vi "DisconnectCameraRslt.vi"(8 "error in (no error)":errorcluster, 11 "CameraTestingUI in":refnum<class "CameraTestingUI.lvclass">) -> (0 "error out":errorcluster, 3 "CameraTestingUI out":refnum<class "CameraTestingUI.lvclass">)   [LabVIEW 2020, in "CameraTestingUI.lvlib" / "CameraTestingUI.lvclass"]
uses:
  CameraTestingUI.lvclass
  CameraTestingUI.lvclass/CameraTestingUI.ctl
  Private/TypeDef/ConnectionStatus.ctl
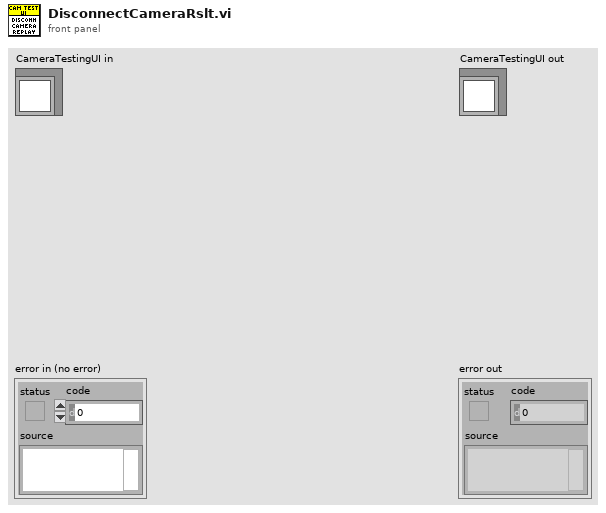
[diagram p1: front panel]
types:
  T1 = enum8{"Enabled", "Disabled", "Disabled and Grayed Out"}
  T2 = typedef "CameraTestingUI.lvlib/CameraTestingUI.lvclass/ConnectionStatus.ctl" = u16
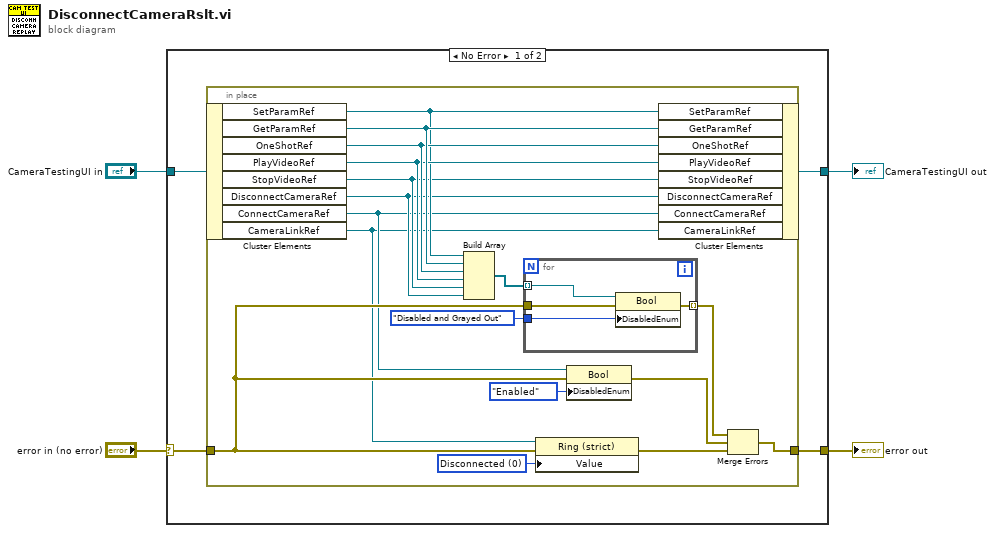
[diagram p0: block diagram]
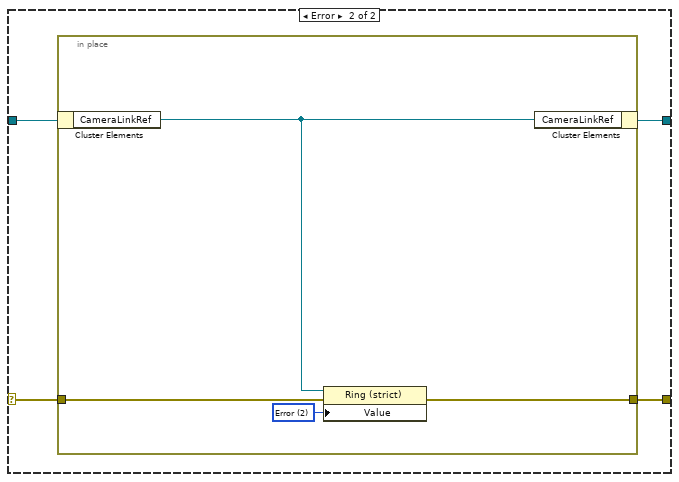
[diagram p2: hidden frame]
diagram:
  n1 = case shown="No Error" "error in (no error)" {
    selector: "error in (no error)" -> [w6 w32]
    tunnel: "CameraTestingUI in" -> [w8 w33]
    tunnel: [w7 w30] -> w3
    tunnel: [w5 w31] -> w1
    frame No Error {
      n2 = in-place {
        in-place-border: w6 -> [w17]
        in-place-border: [w13] -> w5
        w9 = T2 0 items=["Disconnected", "Connected", "Error"] ("Value")
        n3 = in-place-cluster #1(w8) -> ("SetParamRef"=w22:refnum<vi>, "GetParamRef"=w25:refnum<vi>, "OneShotRef"=w24:refnum<vi>, "PlayVideoRef"=w23:refnum<vi>, "StopVideoRef"=w21:refnum<vi>, "DisconnectCameraRef"=w20:refnum<vi>, "ConnectCameraRef"=w12:refnum<vi>, "CameraLinkRef"=w11:refnum<vi>)
        n4 = Build Array(w22, w25, w24, w23, w21, w20) -> (w19:refnum<vi>[])
        n5 = for {
          tunnel: w19 -> [w29] mode=indexing
          tunnel: w17 -> [w28]
          tunnel: [w27] -> w16 mode=indexing
          tunnel: T1."Disabled and Grayed Out" ("Disabled") -> [w26]
          n6 = property class="Bool"(reference=w29, error in=w28, "DisabledEnum"=w26) -> (error out=w27:errorcluster)  [unwired: 1 out]
        }
        n7 = property class="Ring (strict)"(reference=w11, error in=w17, "Value"=w9) -> (error out=w14:errorcluster)  [unwired: 1 out]
        n8 = property class="Bool"(reference=w12, error in=w17, "DisabledEnum"=T1."Enabled" ("Disabled")) -> (error out=w15:errorcluster)  [unwired: 1 out]
        n9 = in-place-cluster #1("SetParamRef"=w22, "GetParamRef"=w25, "OneShotRef"=w24, "PlayVideoRef"=w23, "StopVideoRef"=w21, "DisconnectCameraRef"=w20, "ConnectCameraRef"=w12, "CameraLinkRef"=w11) -> (w7:refnum<class "CameraTestingUI.lvclass">)
        n10 = Merge Errors(w16, w15, w14) -> (w13:errorcluster)
      }
    }
    frame Error {
      n11 = in-place {
        in-place-border: w32 -> [w36]
        in-place-border: [w35] -> w31
        w37 = T2 2 items=["Disconnected", "Connected", "Error", "", ""] ("Value")
        n12 = in-place-cluster #2(w33) -> ("CameraLinkRef"=w34:refnum<vi>)
        n13 = property class="Ring (strict)"(reference=w34, error in=w36, "Value"=w37) -> (error out=w35:errorcluster)  [unwired: 1 out]
        n14 = in-place-cluster #2("CameraLinkRef"=w34) -> (w30:refnum<class "CameraTestingUI.lvclass">)
      }
    }
  }
  "error out" <- w1
  "CameraTestingUI out" <- w3
